vi "WPI_UtilitiesHarvestCommandParams.vi"(11 "Command Params":string[][](array[string])) -> (3 "Strings for Exec Transaction":string[](array[string]))   [LabVIEW 2019]
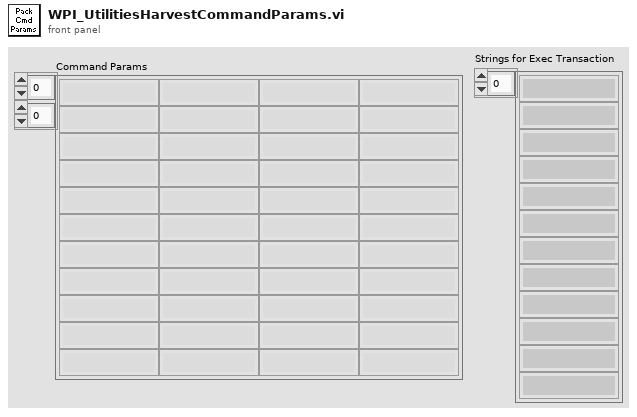
[diagram p1: front panel]
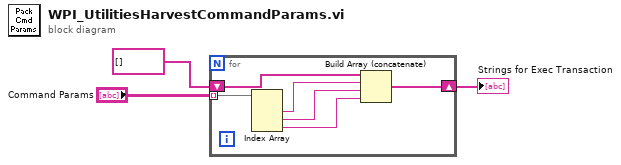
[diagram p0: block diagram]
diagram:
  n1 = for {
    tunnel: "Command Params" -> [w9] mode=indexing
    shift-right: [w7] -> w3
    shift-left: string[] [] -> [w4]
    n2 = Index Array(array=w9) -> (element #1=w8:string, element #2=w6:string, element #3=w5:string)  [unwired: 3 in]
    n3 = Build Array (concatenate)(w4, w8, w6, w5) -> (w7:string[])
  }
  "Strings for Exec Transaction" <- w3
